vi "Initialize Instrument.vi"(8 "error in (no error)":errorcluster, 11 "Instrument.SR7270 in":refnum<class "Instrument.SR7270.lvclass">) -> (0 "error out":errorcluster, 3 "Instrument.SR7270 out":refnum<class "Instrument.SR7270.lvclass">)   [LabVIEW 2016, in "Instrument.SR7270.lvclass"]
uses:
  Instrument.SR7270.lvclass
  Instrument.SR7270.lvclass/Instrument.SR7270.ctl
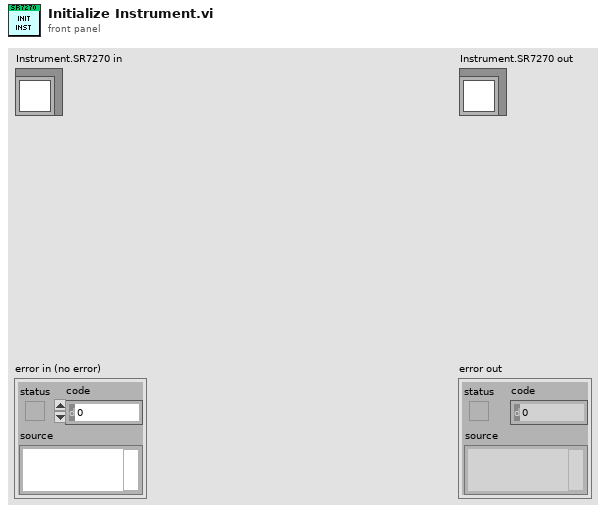
[diagram p1: front panel]
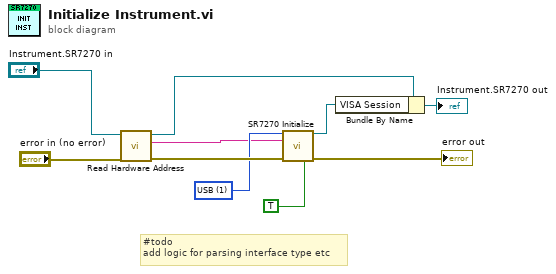
[diagram p0: block diagram]
diagram:
  w4 = u16 1 items=["RS232", "USB", "Ethernet"] ("Interface")
  # "#todo\nadd logic for parsing interface type etc"
  n1 = call-dynamic "Read Hardware Address.vi"("error in (no error)"="error in (no error)", "Instrument in"="Instrument.SR7270 in") -> ("error out"=w7:errorcluster, "Hardware Address"=w1:string, "Instrument out"=w3:refnum<class "Instrument.SR7270.lvclass">)  [unwired: 7 in]
  n2 = call <instrlib>:"SR7270 Initialize.vi"("Interface"=w4, "Serial Number"=w1, "error in (no error)"=w7, "reset"=TRUE) -> ("VISA session"=w6:refnum<visa-resource-name>, "error out"=→"error out":errorcluster)  [unwired: 9 in, 1 out]
  n3 = Bundle By Name(cluster=w3, "VISA Session"=w6) -> (→"Instrument.SR7270 out":refnum<class "Instrument.SR7270.lvclass">)
